vi "PH_Sixpack_Switch.constructor.vi"(0 "name":string, 2 "data in":string, 5 "error in(no error)":errorcluster) -> (14 "i ref out":refnum<vi>, 16 "data out":string, 19 "error out":errorcluster)   [LabVIEW 2014, in "PH_Sixpack_Switch.lvlib"]
doc: "This class is forseen to control easy switches with up to two end position sensors using Beckhoff.\n\nThis class is part of the PHELIX device layer.\n\nauthor: Stefan Götte, GSI\n\nLicense Agreement for this software:\n\nCopyright (C)\nGesellschaft für Schwerionenforschung, GSI\nPlanckstr. 1\n64291 Darmstadt\nGermany\n\nContact: D.Beck@gsi.de \n\nThis program is free software; you can redistribute it and/or modify it under the terms of the \nGNU General Public License as published by the Free Software Foundation; either version 2 of \nthe license, or (at your option) any later version.\n\nThis program is distributed in the hope that it will be useful, but WITHOUT ANY WARRANTY; \nwithout even the implied warranty of MERCHANTABILITY or FITNESS FOR A PARTICULAR PURPOSE. See the GNU General License for more details (http://www.gnu.org).\n\nGesellschaft für Schwerionenforschung, GSI\nPlanckstr. 1, 64291 Darmstadt, Germany\nFor all questions and ideas contact: M.Richter@gsi.de, H.Brand@gsi.de or D.Beck@gsi.de.\nLast update: 16-JUN-2004"
uses:
  PH_Sixpack_Switch.lvlib
  PH_Basics/PH_AxisGUI_BaseClass/PH_AxisGUI_BaseClass.lvlib
  PH_Basics/PH_Class/PH_Class.lvlib
  PH_Basics/PH_PSDBWriter/PH_PSDBWriter.lvlib
  PH_Basics/PH_StatusHandler/PH_StatusHandler.lvlib
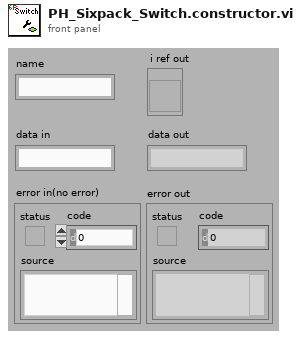
[diagram p1: front panel]
types:
  T1 = enum16{"SetAttribute", "GetAttribute", "CreateAttribute", "DestroyAttribute", "DestroyAllAtributes"}
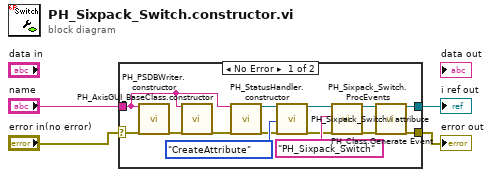
[diagram p0: block diagram]
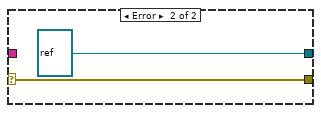
[diagram p2: hidden frame]
diagram:
  n1 = case shown="No Error" "error in(no error)" {
    selector: "error in(no error)" -> [w18 w20]
    tunnel: [w16 refnum<vi> refnum ("i ref out")] -> w4
    tunnel: [w15 w20] -> w3
    tunnel: "name" -> [w6 _]
    frame No Error {
      n2 = call "PH_PSDBWriter.constructor.vi"("name"=w6, "error in"=w18) -> ("error out"=w9:errorcluster)  [unwired: 15 in, 2 out]
      n3 = call "PH_AxisGUI_BaseClass.constructor.vi"("name"=w6, "error in(no error)"=w9) -> ("error out"=w8:errorcluster)  [unwired: 15 in, 2 out]
      n4 = call "PH_StatusHandler.constructor.vi"("name"=w6, "error in(no error)"=w8) -> ("i ref out"=w5:refnum<vi>, "error out"=w7:errorcluster)  [unwired: 15 in, 1 out]
      n5 = call "PH_Sixpack_Switch.i attribute.vi"("VI Refnum"=w5, "Action"=T1."CreateAttribute", "error in (no error)"=w7) -> ("VI Refnum out"=w13:refnum<vi>, "error out"=w11:errorcluster)  [unwired: 14 in, 1 out]
      n6 = call "PH_Class.Generate Event.vi"("i ref in"=w13, "Class"="PH_Sixpack_Switch", "error in (no error)"=w11) -> ("i ref out"=w12:refnum<vi>, "error out"=w10:errorcluster)  [unwired: 15 in]
      n7 = call "PH_Sixpack_Switch.ProcEvents.vi"("i ref in"=w12, "error in (no error)"=w10) -> ("i ref out"=w16:refnum<vi>, "error out"=w15:errorcluster)  [unwired: 16 in]
    }
    frame Error {
    }
  }
  "i ref out" <- w4
  "error out" <- w3
